vi "Header or Footer Same Line.vi"(1 "Header Footer [ ] IN":T1) -> (0 "Header Footer [ ] OUT":T1)   [LabVIEW 2019, in "Exaprom PDF.lvlib"]
doc: "Version 1.0\nDeveloped by Jean-Marc Simard\nCopyright © 2010, Exaprom Inc.\nAll rights reserved.\nLicense: BSD"
uses:
  Exaprom PDF.lvlib
  LV Class/Header and Footer Class/VIs/Controls/Header Footer [ ] V2.ctl
  LV Class/Header and Footer Class/VIs/Controls/Header Footer cluster V2.ctl
  Controls/Header, Footer and Watermark Controls/Header or Footer.ctl
  Controls/Header, Footer and Watermark Controls/Header Footer Type.ctl
  Controls/Header, Footer and Watermark Controls/Header footer horiz alignment.ctl
  Controls/Table Controls/Cell Vertical alignment.ctl
  Controls/Text Controls/Line spacing.ctl
  Controls/Header, Footer and Watermark Controls/Page number.ctl
  Controls/Font Controls/Font complete cluster horizontal.ctl
  Controls/Font Controls/Font size.ctl
  Controls/Font Controls/Font color.ctl
  Controls/Font Controls/Type and encoding.ctl
  Controls/Text Controls/Unicode/Type and run direction.ctl
  C:/work/niobrara_lv/labview pdf writer fixing/DLL/itextsharp.dll
  DLL/itextsharp.dll
  Controls/Header, Footer and Watermark Controls/Header Footer Line.ctl
  General/Stop if it True.vi
  LV Class/Header and Footer Class/Header and Footer Class.lvclass
panel:
  # "X"
  # "Y"
  # "X"
  # "Y"
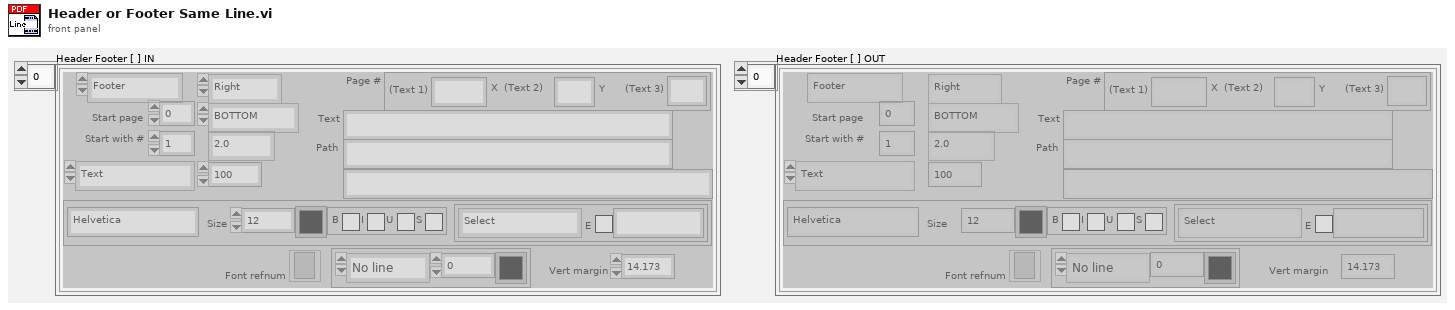
[diagram p1: front panel]
types:
  T1 = typedef "Exaprom PDF.lvlib/Header and Footer Class.lvclass/Header Footer [ ] V2.ctl" = T2[]
  T2 = typedef "Exaprom PDF.lvlib/Header and Footer Class.lvclass/Header Footer cluster V2.ctl" = cluster{"Header or Footer":T3, "Start page":i32, "Start with #":i32, "Type":T4, "Alignment":T5, "Vertical Alignement":T6, "Line spacing":T7, "Image (%)":sgl, "Page #":T8, "Text":string, "Path":string, "Font":T9, "Font refnum":refnum<k24>, "Line":cluster{"Line":T14, "Thickness (points)":sgl, "Colour":T11}, "Vert margin":dbl, "Hyperlink":string}
  T3 = typedef "Exaprom PDF.lvlib/Header or Footer.ctl" = enum16{"Header", "Footer"}
  T4 = typedef "Exaprom PDF.lvlib/Header Footer Type.ctl" = enum16{"Select", "Text", "Text + hyperlink", "Page number", "Image", "Image + hyperlink"}
  T5 = typedef "Exaprom PDF.lvlib/Header footer horiz alignment.ctl" = enum16{"Left", "Center", "Right"}
  T6 = typedef "Exaprom PDF.lvlib/Cell Vertical alignment.ctl" = enum16{"TOP", "MIDDLE", "BOTTOM"}
  T7 = typedef "Exaprom PDF.lvlib/Line spacing.ctl" = enum16{"Select", "1.0", "1.5", "2.0"}
  T8 = typedef "Exaprom PDF.lvlib/Page number.ctl" = cluster{"Text 1":string, "Text 2":string, "Text 3":string}
  T9 = typedef "Exaprom PDF.lvlib/Font complete cluster horizontal.ctl" = cluster{"Name":string, "Size":T10, "Color":T11, "Style":cluster{"Bold":bool, "Italic":bool, "Underline":bool, "Strikeout":bool}, "Type":T12}
  T10 = typedef "Exaprom PDF.lvlib/Font size.ctl" = sgl
  T11 = typedef "Exaprom PDF.lvlib/Font color.ctl" = u32
  T12 = typedef "Exaprom PDF.lvlib/Type and encoding.ctl" = cluster{"Type&direction":T13, "Embedded":bool, "Encoding":string}
  T13 = typedef "Exaprom PDF.lvlib/Type and run direction.ctl" = enum16{"Select", "ASCII", "UTF-16", "UTF-16 (default)", "UTF-16 (LTR)", "UTF-16 (RTL)"}
  T14 = typedef "Exaprom PDF.lvlib/Header Footer Line.ctl" = enum16{"No line", "Horizontal line"}
  T15 = cluster{"Line":T14, "Thickness (points)":sgl, "Colour":T11}
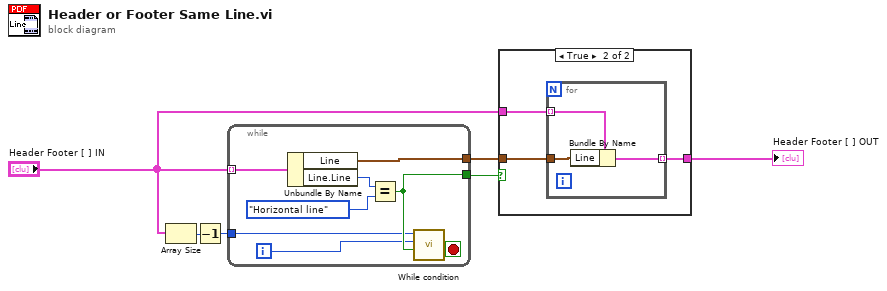
[diagram p0: block diagram]
diagram:
  n1 = Array Size(array="Header Footer [ ] IN") -> (size(s)=w3:i32)
  n2 = Decrement(x=w3) -> (x-1=w1:i32)
  n3 = while {
    tunnel: "Header Footer [ ] IN" -> [w12] mode=indexing
    tunnel: [w9] -> w4
    tunnel: [w11] -> w6
    tunnel: w1 -> [w7]
    i -> [w8]
    stop <- w10 stop-if-true
    n4 = Unbundle By Name(w12) -> ("Line"=w11:T15, "Line.Line"=w14:T14)
    n5 = Equal?(x=w14, y=Header_Footer_Line."Horizontal line") -> (x = y?=w9:bool)
    n6 = call-poly "While condition.vi"("Test"=w9, "i"=w8, "N"=w7) -> ("Action"=w10:bool)  [unwired: 5 out]
  }
  n7 = case shown="True" w4 {
    tunnel: "Header Footer [ ] IN" -> [w15 w18]
    tunnel: w6 -> [_ w17]
    tunnel: [w15 w16] -> w5
    frame False {
    }
    frame True {
      n8 = for {
        tunnel: w18 -> [w21] mode=indexing
        tunnel: w17 -> [w20]
        tunnel: [w19] -> w16 mode=indexing
        n9 = Bundle By Name(cluster=w21, "Line"=w20) -> (w19:T2)
      }
    }
  }
  "Header Footer [ ] OUT" <- w5
